vi "FVI_DirectionAutonome.vi"(10 "Direction":dbl, 11 "vitesse":dbl) -> (2 "x":dbl, 3 "y":dbl)   [LabVIEW 2018]
panel:
  out "sqrt(x)":dbl
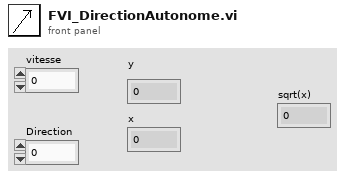
[diagram p1: front panel]
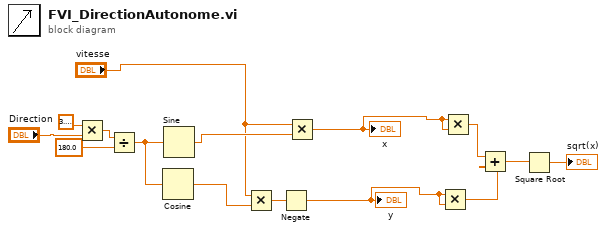
[diagram p0: block diagram]
diagram:
  n1 = Multiply(x=3.141592653589793, y="Direction") -> (x*y=w4:dbl)
  n2 = Divide(x=w4, y=180.0) -> (x/y=w1:dbl)
  n3 = Cosine(x=w1) -> (cos(x)=w15:dbl)
  n4 = Sine(x=w1) -> (sin(x)=w13:dbl)
  n5 = Multiply(x="vitesse", y=w15) -> (x*y=w14:dbl)
  n6 = Negate(x=w14) -> (-x=w10:dbl)
  "y" <- w10
  n7 = Multiply(x="vitesse", y=w13) -> (x*y=w11:dbl)
  "x" <- w11
  n8 = Multiply(x=w10, y=w10) -> (x*y=w8:dbl)
  n9 = Multiply(x=w11, y=w11) -> (x*y=w9:dbl)
  n10 = Add(x=w9, y=w8) -> (x+y=w7:dbl)
  n11 = Square Root(x=w7) -> (sqrt(x)=→"sqrt(x)":dbl)
